vi "SysDef.Property.Get.DependentFile.vi"(8 "error in (no error)":errorcluster, 10 "Property Name":string, 11 "nodeID":u64) -> (0 "error out":errorcluster, 1 "Value":T1, 3 "nodeID out":u64, 4 "Found?":bool)   [LabVIEW 2024, in "Advanced System Definition.lvlib"]
uses:
  SysDef API/Advanced System Definition.lvlib
  C:/NetCore/niveristand-custom-device-development-tools/advanced-sysdef-api/Source/_SubVIs/SysDef.Property.Get.DependentFile.vi/NationalInstruments.VeriStand.SystemDefinitionAPI
  NationalInstruments.VeriStand.SystemDefinitionAPI
  <vilib>/NI VeriStand/Custom Device API/Custom Device API.lvlib
  <vilib>/NI VeriStand/Custom Device API/Get Item Property (Dependent File).vi
  _Types/Property.DependentFile.ctl
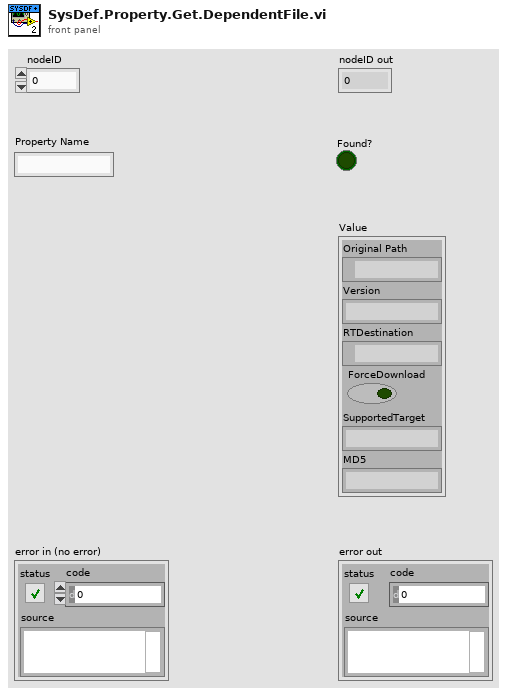
[diagram p1: front panel]
types:
  T1 = typedef "Advanced System Definition.lvlib/Property.DependentFile.ctl" = cluster{"Original Path":path, "Version":string, "RTDestination":path, "ForceDownload":bool, "SupportedTarget":string, "MD5":string}
  T2 = typedef "Custom Device API.lvlib/Custom Device Item Ref.ctl" = u64
  T3 = typedef "Custom Device API.lvlib/Dependent File Optional Info.ctl" = cluster{"Version":string, "RTDestination":path, "ForceDownload":bool, "SupportedTarget":string, "MD5":string}
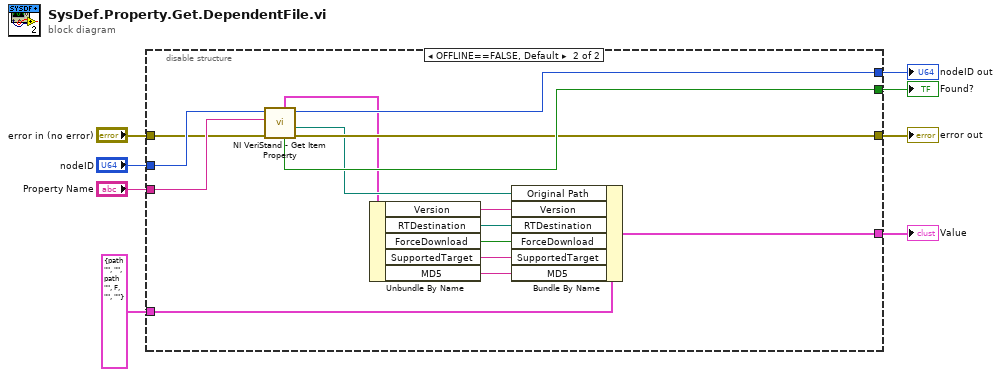
[diagram p0: block diagram]
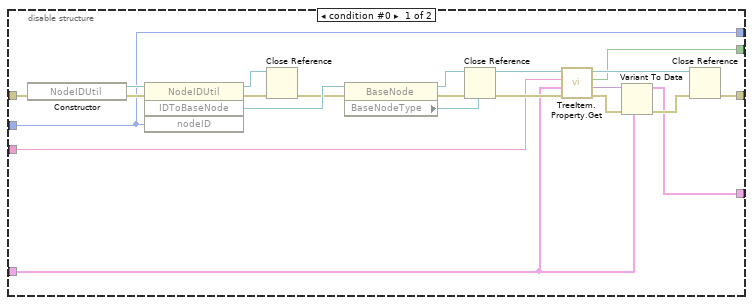
[diagram p2: hidden frame]
diagram:
  n1 = disable-structure shown="OFFLINE==FALSE, Default" {
    disable-tunnel: "error in (no error)" -> [w22 w42]
    disable-tunnel: "nodeID" -> [w9 w43]
    disable-tunnel: [w17 w40] -> w6
    disable-tunnel: "Property Name" -> [w16 w44]
    disable-tunnel: [w12 w41] -> w4
    disable-tunnel: T1 {"Original Path"=path "", "Version"="", "RTDestination"=path "", "ForceDownload"=FALSE, "SupportedTarget"="", "MD5"=""} ("Value") -> [w11 w38]
    disable-tunnel: [w10 w36] -> w2
    disable-tunnel: [w9 w39] -> w1
    frame condition #0 {
      n2 = constructor class="NodeIDUtil"(error in=w22) -> (reference out=w29:refnum<k24>, error out=w28:errorcluster)  [unwired: 2 in, 1 out]
      n3 = invoke class="NodeIDUtil" method="IDToBaseNode"(reference=w29, error in=w28, "nodeID"=w9) -> (reference out=w23:refnum<k24>, error out=w25:errorcluster, "IDToBaseNode"=w27:refnum<k24>)  [unwired: 1 in, 1 out]
      n4 = Close Reference(reference=w23, error in (no error)=w25) -> (error out=w24:errorcluster)
      n5 = property class="BaseNode"(reference=w27, error in=w24) -> (reference out=w21:refnum<k24>, error out=w20:errorcluster, "BaseNodeType"=w26:refnum<k24>)
      n6 = Close Reference(reference=w21, error in (no error)=w20) -> (error out=w19:errorcluster)
      n7 = call "TreeItem.Property.Get.vi"("error in (no error)"=w19, "Default Value"=w11, "Property Name"=w16, "NationalInstruments.VeriStand.SystemStorage.BaseNodeType"=w26) -> ("error out"=w14:errorcluster, "Variant"=w15:variant, "Found?"=w12:bool, "NationalInstruments.VeriStand.SystemStorage.BaseNodeType"=w18:refnum<k39>)  [unwired: 4 in]
      n8 = Variant To Data(error in=w14, type=w11, Variant=w15) -> (data=w10:T1, error out=w13:errorcluster)
      n9 = Close Reference(reference=w18, error in (no error)=w13) -> (error out=w17:errorcluster)
    }
    frame condition #1 (active) {
      n10 = call-poly <vilib>:"NI VeriStand - Get Item Property.vi"("error in (no error)"=w42, "Property Name"=w44, "Item Ref in"=w43) -> ("error out"=w40:errorcluster, "Path"=w37:path, "Item Ref out"=w39:T2, "Found"=w41:bool, "OptionalInfo"=w35:T3)  [unwired: 4 in]
      n11 = Unbundle By Name(w35) -> ("Version"=w34:string, "RTDestination"=w33:path, "ForceDownload"=w32:bool, "SupportedTarget"=w31:string, "MD5"=w30:string)
      n12 = Bundle By Name(cluster=w38, "Original Path"=w37, "Version"=w34, "RTDestination"=w33, "ForceDownload"=w32, "SupportedTarget"=w31, "MD5"=w30) -> (w36:T1)
    }
  }
  "nodeID out" <- w1
  "error out" <- w6
  "Value" <- w2
  "Found?" <- w4
